vi "Img Get Pic Img By Index.vi"(8 "error in (no error)":errorcluster, 9 "Pic Num":u32, 10 "Img Json Data":T2[](array[typedef]), 11 "Img Data":cluster{"image data":T1, "bitmap":u32[][]}[](array[cluster])) -> (0 "error out":errorcluster, 1 "Found?":bool, 2 "frames":T3, 3 "Img Data Indexed":cluster{"image data":T1, "bitmap":u32[][]})   [LabVIEW 2018, in "Main Panel.lvlib" / "Main Panel.lvclass"]
uses:
  Main Panel.lvclass
  Image Json Parser/Img Json Frames.ctl
  Image Json Parser/Img Json Data.ctl
  Image Json Parser/Img Json Meta.ctl
  <vilib>/picture/picture.llb/imagedata.ctl
  Image Json Parser/Image Json Parser.lvclass
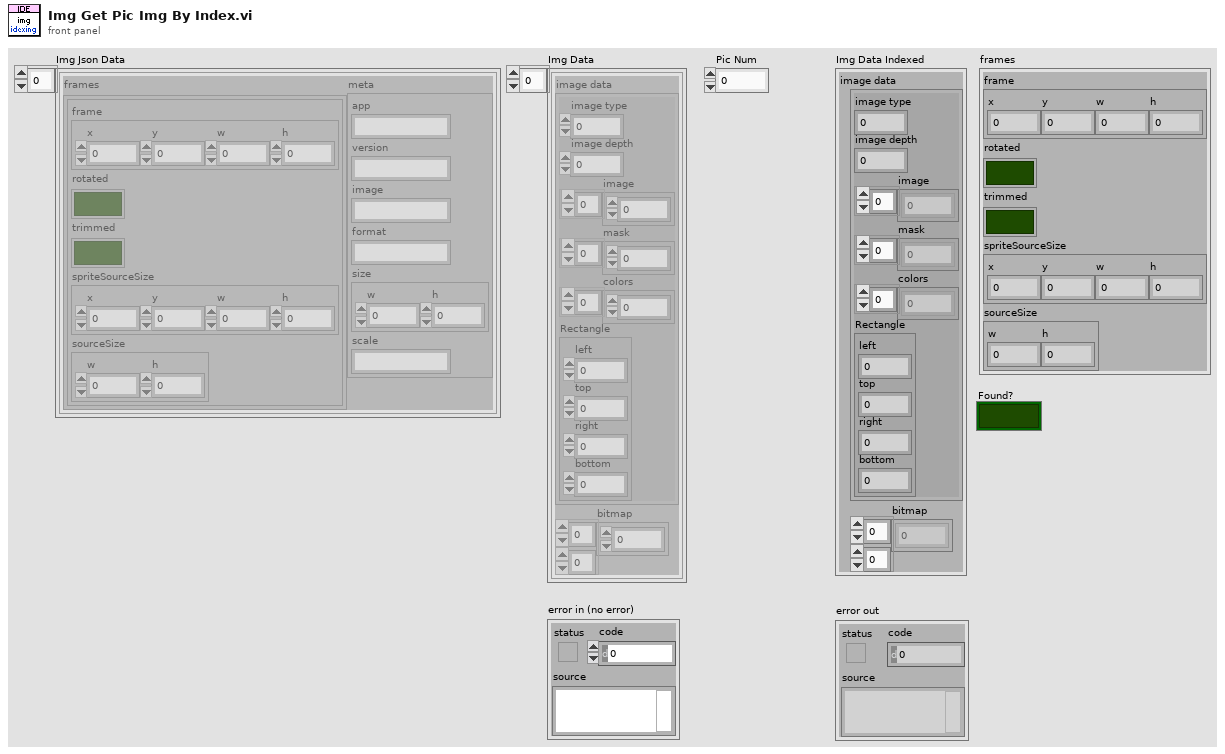
[diagram p1: front panel]
types:
  T1 = typedef "imagedata.ctl" = cluster{"image type":i32, "image depth":i32, "image":u8[], "mask":u8[], "colors":u32[], "Rectangle":cluster{"left":i16, "top":i16, "right":i16, "bottom":i16}}
  T2 = typedef "Image Json Parser.lvclass/Img Json Data.ctl" = cluster{"frames":T3[], "meta":T4}
  T3 = typedef "Image Json Parser.lvclass/Img Json Frames.ctl" = cluster{"frame":cluster{"x":i32, "y":i32, "w":i32, "h":i32}, "rotated":bool, "trimmed":bool, "spriteSourceSize":cluster{"x":i32, "y":i32, "w":i32, "h":i32}, "sourceSize":cluster{"w":i32, "h":i32}}
  T4 = typedef "Image Json Parser.lvclass/Img Json Meta.ctl" = cluster{"app":string, "version":string, "image":string, "format":string, "size":cluster{"w":i32, "h":i32}, "scale":string}
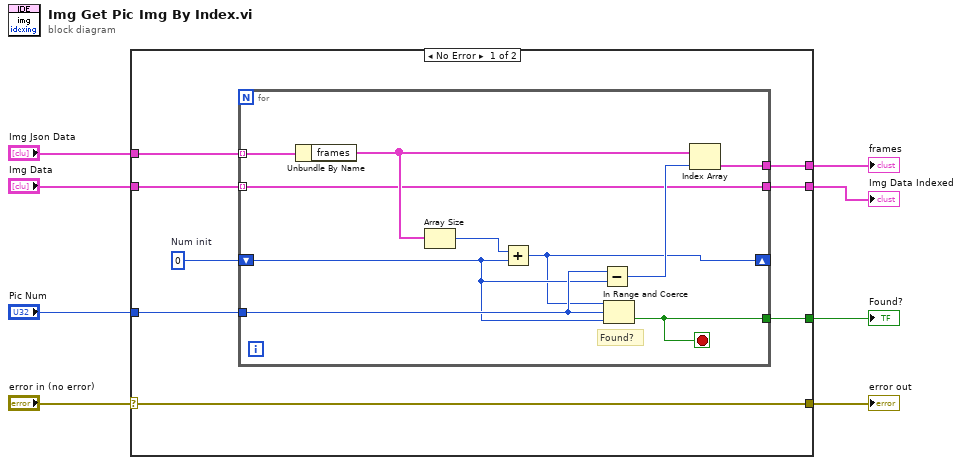
[diagram p0: block diagram]
diagram:
  n1 = case shown="No Error" "error in (no error)" {
    selector: "error in (no error)" -> [w16 w27]
    tunnel: [w16 w27] -> w7
    tunnel: "Pic Num" -> [w15 _]
    tunnel: [w13 _] -> w5
    tunnel: [w12 _] -> w4
    tunnel: "Img Json Data" -> [w11 _]
    tunnel: "Img Data" -> [w10 _]
    tunnel: [w9 _] -> w1
    frame No Error {
      w14 = 0  # Num init
      n2 = for {
        tunnel: w11 -> [w26] mode=indexing
        shift-right: [w20] -> _
        shift-left: w14 -> [w22]
        tunnel: w15 -> [w23]
        tunnel: [w19] -> w13
        tunnel: [w18] -> w12
        tunnel: w10 -> [w17] mode=indexing
        tunnel: [w17] -> w9
        stop <- w18 stop-if-true
        # "Found?"
        n3 = Unbundle By Name(w26) -> ("frames"=w24:T3[])
        n4 = Array Size(array=w24) -> (size(s)=w25:i32)
        n5 = Add(x=w25, y=w22) -> (x+y=w20:i32)
        n6 = Subtract(x=w23, y=w22) -> (x-y=w21:u32)
        n7 = In Range and Coerce(upper limit=w20, x=w23, lower limit=w22) -> (In Range?=w18:bool)  [unwired: 1 out]
        n8 = Index Array(array=w24, index=w21) -> (element=w19:T3)
      }
    }
    frame Error {
    }
  }
  "error out" <- w7
  "frames" <- w5
  "Found?" <- w4
  "Img Data Indexed" <- w1
